vi "fxp32_16-to-int.vi"(10 "FXP32_16":fxp<+/-,32,16>) -> (2 "32bit integer":i32)   [LabVIEW 2018]
uses:
  <vilib>/rvi/FXPMathLib/FxpInterpret/XNode/nifxpmath_Interpret.xnode
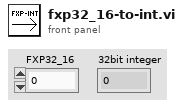
[diagram p1: front panel]
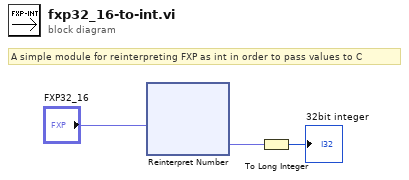
[diagram p0: block diagram]
diagram:
  # "A simple module for reinterpreting FXP as int in order to pass values to C"
  n1 = xnode "Reinterpret Number"("x"="FXP32_16") -> ("y"=w2:fxp<+/-,32,32>)
  n2 = To Long Integer(number=w2) -> (32bit integer=→"32bit integer":i32)
